vi "GFBuildFastTriggerWaveForm.vi"(0 "task in":refnum<k21>="PCIE-FastFire", 1 "Trigger Width":dbl=4e-05, 2 "Special Trigger Width":dbl=4e-05, 3 "Special Trig index":u32, 5 "error in":errorcluster, 6 "Enable Array":bool[](array[boolean]), 7 "Chan Delays":dbl[](array[numeric])=[0.0001, 0.0003, 0.0005, 0.0007, 0.0013] format="%.6f", 9 "Special Trigger Width 2":dbl=4e-05, 10 "Special Trigger Width 3":dbl=4e-05, 11 "Special Trig index 2":u32, 12 "Special Trig index 3":u32) -> (14 "task out":refnum<k21>, 16 "Digital Waveform Graph":digitalwaveform[](graph), 19 "error out":errorcluster)   [LabVIEW 2009]
doc: "This subVI creates an N dimensional Boolean array based on the number of channels in the task."
uses:
  <vilib>/Waveform/DWDTOps.llb/DWDT Boolean Array to Digital.vi
  Program Files (x86)/National Instruments/LabVIEW 2009/resource/objmgr/daqmx.rc
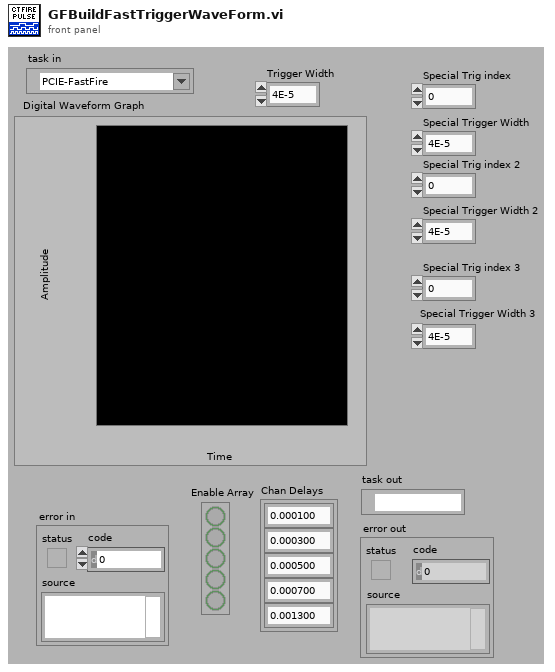
[diagram p1: front panel]
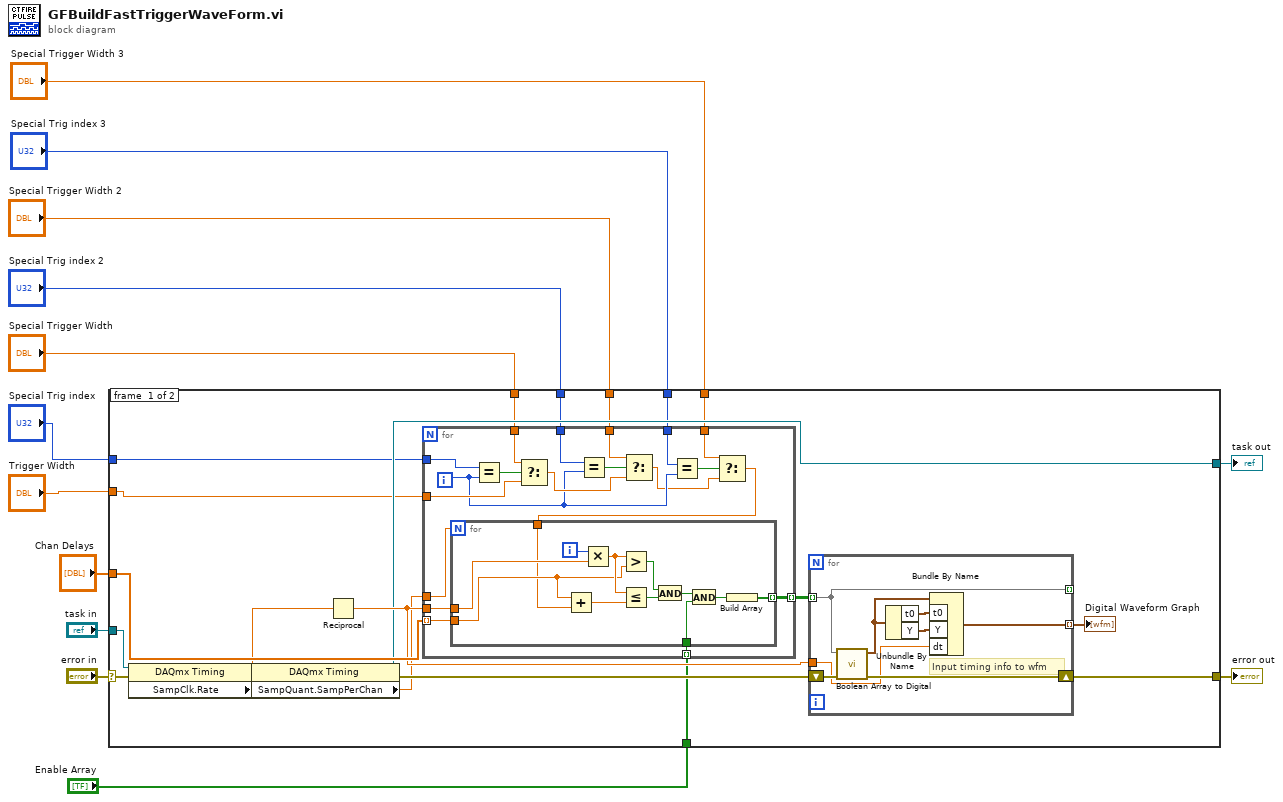
[diagram p0: block diagram]
diagram:
  n1 = case shown="No Error" "error in" {
    selector: "error in" -> [w28 w74]
    tunnel: "task in" -> [w29 w75]
    tunnel: [w24 w75] -> w12
    tunnel: [w33 w74] -> w10
    tunnel: "Chan Delays" -> [w32 _]
    tunnel: "Enable Array" -> [w21 _]
    tunnel: "Trigger Width" -> [w20 _]
    tunnel: "Special Trig index" -> [w19 _]
    tunnel: "Special Trigger Width" -> [w18 _]
    tunnel: "Special Trig index 2" -> [w17 _]
    tunnel: "Special Trigger Width 2" -> [w16 _]
    tunnel: "Special Trig index 3" -> [w15 _]
    tunnel: "Special Trigger Width 3" -> [w14 _]
    frame #0 {
      n2 = property class="DAQmx Timing"(reference=w29, error in=w28) -> (reference out=w26:refnum<k21>, error out=w25:errorcluster, "SampClk.Rate"=w27:dbl)
      n3 = property class="DAQmx Timing"(reference=w26, error in=w25) -> (reference out=w24:refnum<k21>, error out=w23:errorcluster, "SampQuant.SampPerChan"=w22:dbl)
      n4 = Reciprocal(x=w27) -> (1/x=w31:dbl)
      n5 = for {
        tunnel: [w58] -> w34 mode=indexing
        tunnel: w32 -> [w61] mode=indexing
        tunnel: w31 -> [w60]
        tunnel: w22 -> [w59]
        tunnel: w21 -> [w57] mode=indexing
        tunnel: w20 -> [w53]
        tunnel: w19 -> [w56]
        tunnel: w18 -> [w54]
        tunnel: w17 -> [w51]
        tunnel: w16 -> [w50]
        tunnel: w15 -> [w47]
        tunnel: w14 -> [w46]
        i -> [w45]
        n6 = Equal?(x=w56, y=w45) -> (x = y?=w55:bool)
        n7 = Select(t=w54, s=w55, f=w53) -> (s? t:f=w49:dbl)
        n8 = Equal?(x=w51, y=w45) -> (x = y?=w52:bool)
        n9 = Select(t=w50, s=w52, f=w49) -> (s? t:f=w44:dbl)
        n10 = Equal?(x=w47, y=w45) -> (x = y?=w48:bool)
        n11 = Select(t=w46, s=w48, f=w44) -> (s? t:f=w43:dbl)
        n12 = for {
          N: w59 -> [_]
          tunnel: w61 -> [w71]
          tunnel: w60 -> [w73]
          tunnel: [w66] -> w58 mode=indexing
          tunnel: w57 -> [w63]
          tunnel: w43 -> [w62]
          i -> [w65]
          n13 = Add(x=w71, y=w62) -> (x+y=w70:dbl)
          n14 = Multiply(x=w65, y=w73) -> (x*y=w72:dbl)
          n15 = Greater?(x=w72, y=w71) -> (0:w69:bool)
          n16 = Less Or Equal?(x=w72, y=w70) -> (x <= y?=w68:bool)
          n17 = And(x=w69, y=w68) -> (x .and. y?=w67:bool)
          n18 = And(x=w67, y=w63) -> (x .and. y?=w64:bool)
          n19 = Build Array(w64) -> (w66:bool[])
        }
      }
      n20 = for {
        shift-right: [w42] -> w33
        shift-left: w23 -> [w41]
        tunnel: w34 -> [w35] mode=indexing
        tunnel: [w36] -> w30 mode=indexing
        tunnel: w31 -> [w38]
        tunnel: [w35] -> _ mode=indexing
        # "Input timing info to wfm"
        n21 = call-poly <vilib>:"Boolean Array to Digital.vi"("error in (no error)"=w41, "boolean array"=w35) -> ("error out"=w42:errorcluster, "digital waveform"=w37:digitalwaveform)  [unwired: 8 in]
        n22 = Unbundle By Name(w37) -> ("t0"=w40:timestamp, "Y"=w39:digitaldata)
        n23 = Bundle By Name(cluster=w37, "t0"=w40, "Y"=w39, "dt"=w38) -> (w36:digitalwaveform)
      }
      "Digital Waveform Graph" <- w30
    }
    frame #1 {
    }
  }
  "error out" <- w10
  "task out" <- w12
